vi "manual_ws_conn_parser.vi"() -> ()   [LabVIEW 2013]
uses:
  <vilib>/Intelligent Energy/WebSockets API/WebSockets/WebSockets.lvlib
panel:
  out "axes":sgl[](array[numeric])
  out "buttons":i32[](array[numeric])
  out "incomming\nmessage":T1
  out "value":T1
  in  "?":T1
  out "String":string
  in  "stop":bool
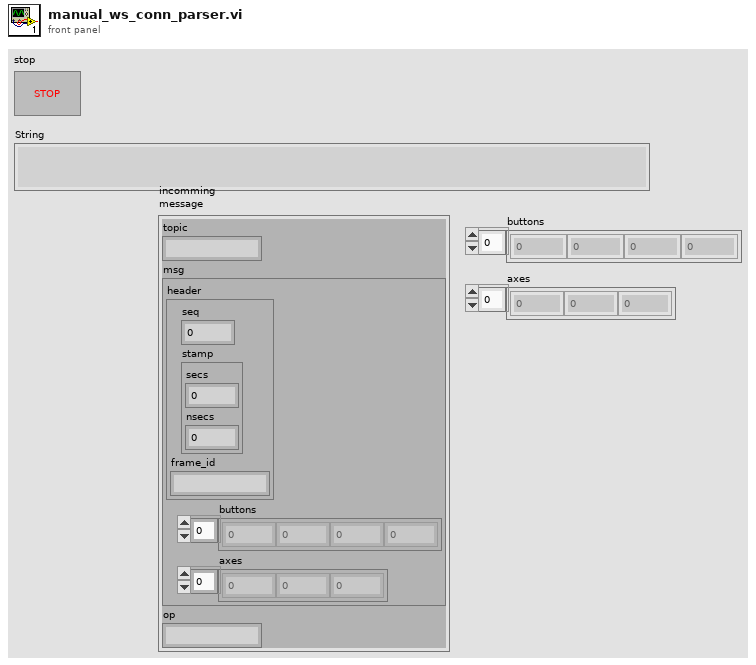
[diagram p1: front panel]
types:
  T1 = cluster{"topic":string, "msg":cluster{"header":cluster{"seq":u32, "stamp":cluster{"secs":u32, "nsecs":i32}, "frame_id":string}, "buttons":i32[], "axes":sgl[]}, "op":string}
  T2 = enum16{"Standard", "Buffered", "CRLF", "Immediate"}
  T3 = cluster{"header":cluster{"seq":u32, "stamp":cluster{"secs":u32, "nsecs":i32}, "frame_id":string}, "buttons":i32[], "axes":sgl[]}
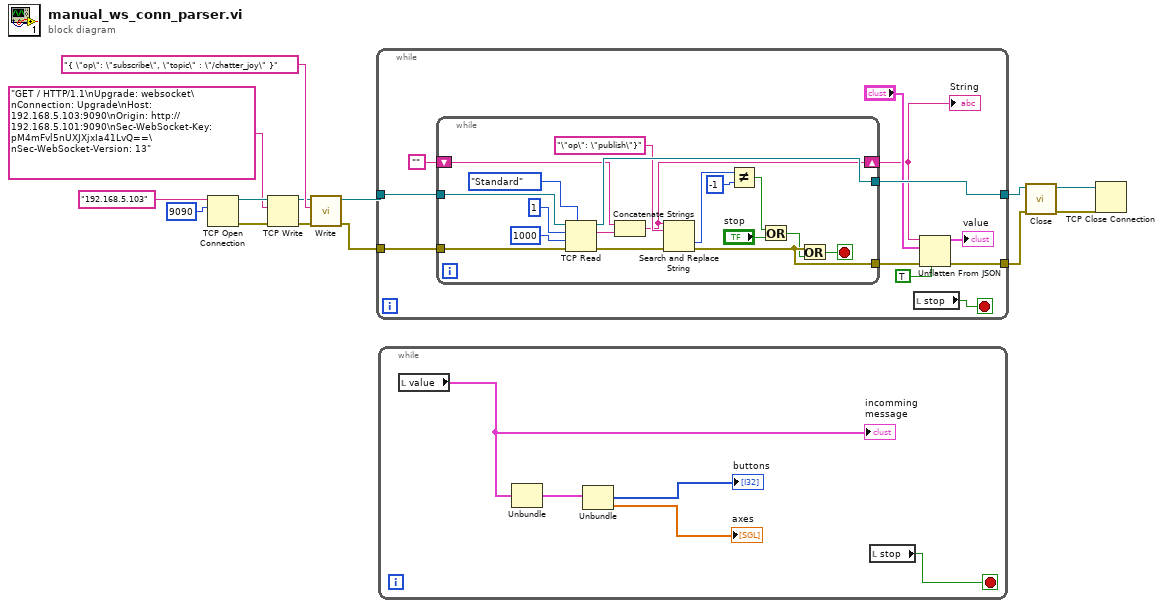
[diagram p0: block diagram]
diagram:
  n1 = TCP Open Connection(address="192.168.5.103", remote port or service name=u16 9090) -> (connection ID=w12:refnum<k5>, error out=w10:errorcluster)  [unwired: 3 in]
  n2 = TCP Write(connection ID=w12, data in="GET / HTTP/1.1\nUpgrade: websocket\nConnection: Upgrade\nHost: 192.168.5.103:9090\nOrigin: http://192.168.5.101:9090\nSec-WebSocket-Key: pM4mFvl5nUXJXjxIa41LvQ==\nSec-WebSocket-Version: 13", error in (no error)=w10) -> (connection ID out=w6:refnum<k5>, error out=w5:errorcluster)  [unwired: 1 in, 1 out]
  n3 = call <vilib>:"Write.vi"("error in (no error)"=w5, "Data"="{ \"op\": \"subscribe\", \"topic\" : \"/chatter_joy\" }", "WebSocket Connection in"=w6) -> ("error out"=w1:errorcluster, "WebSocket Connection out"=w2:refnum<k5>)  [unwired: 7 in]
  n4 = while {
    tunnel: [w25] -> w4
    tunnel: [w19] -> w3
    tunnel: w2 -> [w24]
    tunnel: w1 -> [w23]
    stop <- w22 stop-if-true
    n5 = while {
      tunnel: [w41] -> w25
      tunnel: [w34] -> w20
      tunnel: w24 -> [w42]
      tunnel: w23 -> [w37]
      shift-right: [w26] -> w17
      shift-left: "" -> [w28]
      stop <- w43 stop-if-true
      n6 = TCP Read(connection ID=w42, bytes to read=1, error in (no error)=w37, 7:T2."Standard" ("mode (standard)"), 9:1000 ("timeout ms (25000)")) -> (connection ID out=w41:refnum<k5>, data out=w27:string, error out=w35:errorcluster)
      n7 = Concatenate Strings(w28, w27) -> (w26:string)
      n8 = Search and Replace String(input string=w26, search string="\"op\": \"publish\"}", error in=w35) -> (offset past replacement=w31:i32, error out=w34:errorcluster)  [unwired: 5 in, 2 out]
      n9 = Not Equal?(x=w31, y=-1) -> (x != y?=w33:bool)
      n10 = Or(x=w33, y="stop") -> (x .or. y?=w29:bool)
      n11 = Or(x=w34, y=w29) -> (x .or. y?=w43:bool)
    }
    "String" <- w17
    n12 = local read "stop"() -> (w22:bool)
    n13 = Unflatten From JSON(JSON string=w17, type and defaults="?", default null elements? (F)=TRUE, error in (no error)=w20) -> (value=→"value":T1, error out=w19:errorcluster)  [unwired: 3 in]
  }
  n14 = while {
    stop <- w48 stop-if-true
    n15 = local read "value"() -> (w47:T1)
    "incomming\nmessage" <- w47
    n16 = Unbundle(w47) -> ("msg"=w46:T3)  [unwired: 2 out]
    n17 = Unbundle(w46) -> ("buttons"=→"buttons":i32[], "axes"=→"axes":sgl[])  [unwired: 1 out]
    n18 = local read "stop"() -> (w48:bool)
  }
  n19 = call <vilib>:"Close.vi"("error in (no error)"=w3, "WebSocket Connection in"=w4) -> ("error out"=w7:errorcluster, "WebSocket Connection in"=w8:refnum<k5>)  [unwired: 8 in]
  n20 = TCP Close Connection(connection ID=w8, error in (no error)=w7) -> ()  [unwired: 1 in, 2 out]
